vi "Get Driver List - Single Converter.vi"(11 "error in":errorcluster) -> (15 "error out":errorcluster)   [LabVIEW 2021, in "Converter.lvlib"]
uses:
  Converter.lvlib
  <vilib>/Utility/traverseref.llb/TRef TravTarget.ctl
  <vilib>/Utility/traverseref.llb/VI Scripting - Traverse.lvlib
  Converter Reusables/Converter Reusables.lvlib
  Path Functions/Path Functions.lvlib
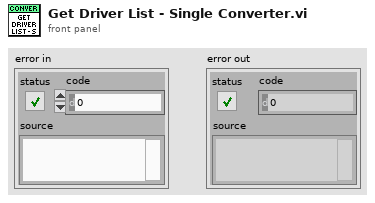
[diagram p1: front panel]
types:
  T1 = typedef "TRef TravTarget.ctl" = enum16{"FP", "BD", "Other"}
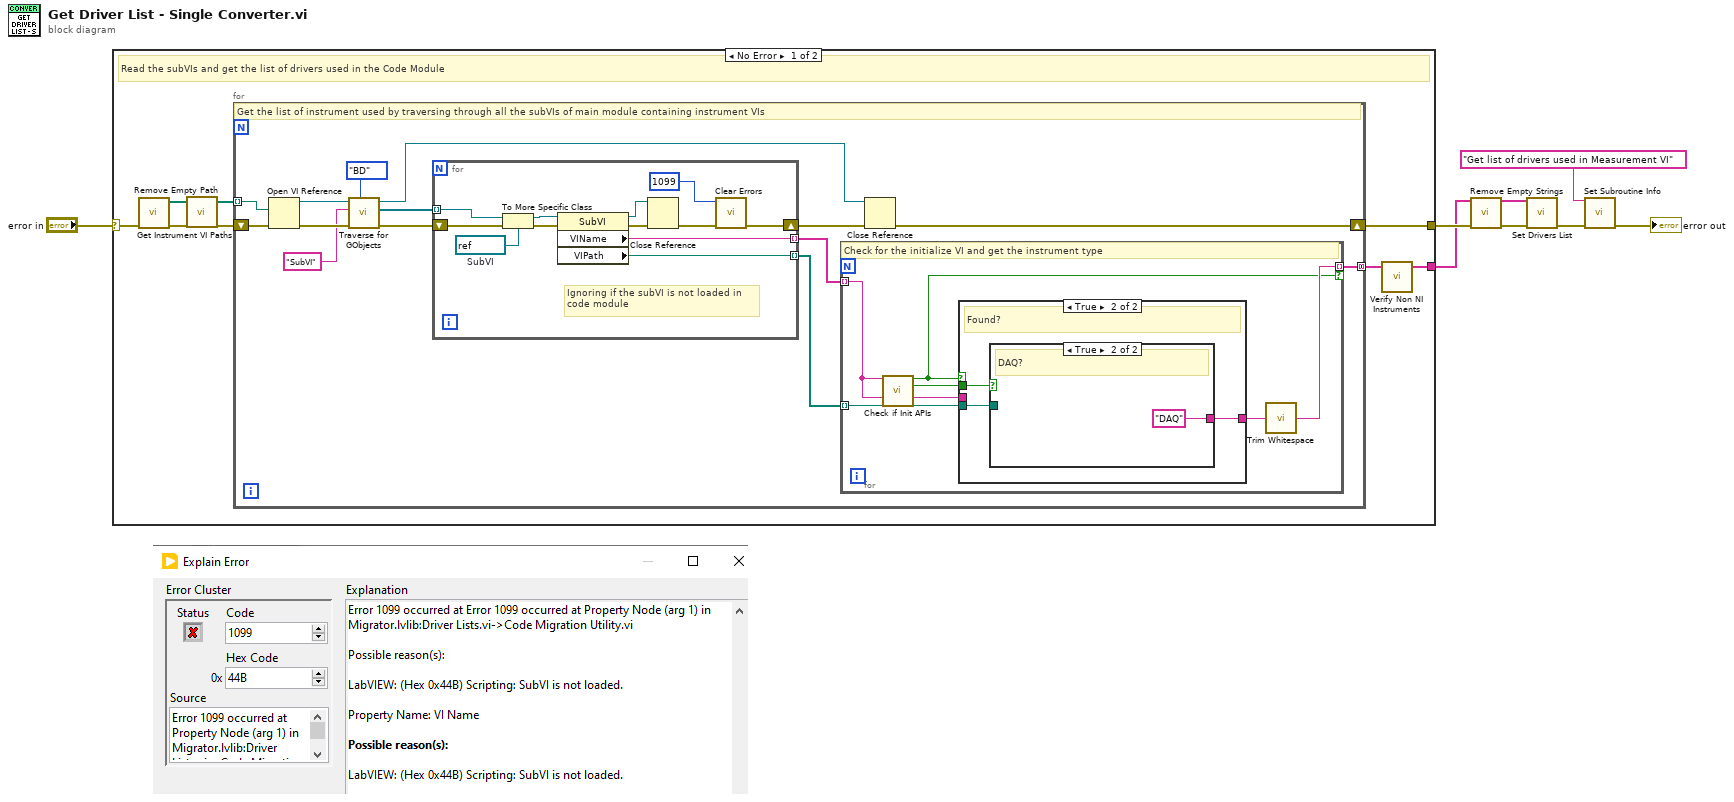
[diagram p0: block diagram]
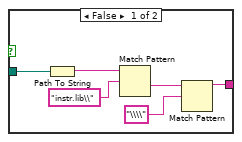
[diagram p3: hidden frame]
diagram:
  n1 = case shown="No Error" "error in" {
    selector: "error in" -> [w13 w57]
    tunnel: [w9 w57] -> w6
    tunnel: [w10 _] -> w2
    frame No Error {
      # "Read the subVIs and get the list of drivers used in the Code Module"
      n2 = call "Get Instrument VI Paths.vi"("error in"=w13) -> ("error out"=w12:errorcluster, "instr vi paths[]"=w14:path[])  [unwired: 9 in]
      n3 = call "Remove Empty Path.vi"("instr vi paths in"=w14) -> ("instr vi paths out"=w8:path[])  [unwired: 4 in]
      n4 = for {
        tunnel: w8 -> [w23] mode=indexing
        tunnel: [w19] -> w11 mode=concatenating
        shift-right: [w17] -> w9
        shift-left: w12 -> [w22]
        # "Get the list of instrument used by traversing through all the subVIs of main module containing instrument VIs"
        n5 = Open VI Reference(vi path=w23, error in (no error)=w22) -> (vi reference=w18:refnum<vi>, error out=w26:errorcluster)  [unwired: 4 in]
        n6 = call <vilib>:"Traverse for GObjects.vi"("Traverse Target"=TRef_TravTarget."BD", "error in (no error)"=w26, "Class Name"="SubVI", "VI Refnum"=w18) -> ("error out"=w28:errorcluster, "References"=w27:refnum<vi>[], "dup VI Refnum"=w15:refnum<vi>)  [unwired: 4 in, 1 out]
        n7 = for {
          tunnel: w27 -> [w55] mode=indexing
          tunnel: [w51] -> w21 mode=indexing
          tunnel: [w50] -> w20 mode=indexing
          shift-right: [w46] -> w16
          shift-left: w28 -> [w54]
          w56 = refnum<vi> refnum  # SubVI
          # "Ignoring if the subVI is not loaded in\ncode module"
          n8 = To More Specific Class(target class=w56, reference=w55, error in=w54) -> (specific class reference=w53:refnum<vi>, error out=w52:errorcluster)
          n9 = property class="SubVI"(reference=w53, error in=w52) -> (reference out=w49:refnum<vi>, error out=w48:errorcluster, "VIName"=w51:string, "VIPath"=w50:path)
          n10 = Close Reference(reference=w49, error in (no error)=w48) -> (error out=w47:errorcluster)
          n11 = call <vilib>:"Clear Errors.vi"("error in (no error)"=w47, "specific error code to clear (0: all)"=1099) -> ("error out"=w46:errorcluster)  [unwired: 4 in, 1 out]
        }
        n12 = for {
          tunnel: w21 -> [w30] mode=indexing
          tunnel: w20 -> [w34] mode=indexing
          tunnel: [w33] -> w19 mode=indexing if=w31
          # "Check for the initialize VI and get the instrument type"
          n13 = call "Check if Init APIs.vi"("vi name"=w30) -> ("instrument driver found?"=w31:bool, "daq?"=w29:bool)  [unwired: 13 in]
          n14 = case shown="True" w31 {
            tunnel: w34 -> [_ w37]
            tunnel: [_ w36] -> w32
            tunnel: w30 -> [_ _]
            tunnel: w29 -> [_ w35]
            frame False {
            }
            frame True {
              # "Found?"
              n15 = case shown="True" w35 {
                tunnel: w37 -> [w39 _]
                tunnel: [w38 "DAQ"] -> w36
                frame False {
                  n16 = Path To String(path=w39) -> (string=w40:string)
                  n17 = Match Pattern(string=w40, regular expression="instr.lib\\") -> (after substring=w42:string)  [unwired: 1 in, 3 out]
                  n18 = Match Pattern(string=w42, regular expression="\\\\") -> (before substring=w38:string)  [unwired: 1 in, 3 out]
                }
                frame True {
                  # "DAQ?"
                }
              }
            }
          }
          n19 = call <vilib>:"Trim Whitespace.vi"("string"=w32) -> ("trimmed string"=w33:string)  [unwired: 1 in]
        }
        n20 = Close Reference(reference=w15, error in (no error)=w16) -> (error out=w17:errorcluster)
      }
      n21 = call "Verify Non NI Instruments.vi"("instrument types in"=w11) -> ("instrument types out"=w10:string[])  [unwired: 4 in]
    }
    frame Error {
    }
  }
  n22 = call "Remove Empty Strings.vi"("instrument types in"=w2) -> ("instrument types out"=w1:string[])  [unwired: 14 in]
  n23 = call "Set Drivers List.vi"("name"=w1, "error in"=w6) -> ("error out"=w5:errorcluster)  [unwired: 13 in]
  n24 = call "Set Subroutine Info.vi"("subroutine in"="Get list of drivers used in Measurement VI" ("Subroutine In"), "error in"=w5) -> ("error out"=→"error out":errorcluster)  [unwired: 13 in]
